vi "OE2031&OE2041_Configure Demodulation.vi"(7 "OE2041_Configure Demodulator":T1={"A"=1, "F1"=1.0, "B"=1, "F2"=1.0, "Demodulator"=1, "Mode"=0, "Arbitrary Frequency"=1000.0, "Harmonic"=1, "Instrument Mode "=8} {"Instrument Mode" items=["OE2031-10M"=6, "OE2041-30M"=7, "OE2041-60M"=8]; "Harmonic" min=1 max=32767; "Arbitrary Frequency" min=1e-05 max=60000000.0 format="%#.3f"; "Mode" items=["Harm", "Arb_Freq", "Equation"]; "Demodulator" items=["1", "2", "3"]; "F2" min=1e-05 max=60000000.0 format="%#.3g"; "B" min=-32767; "F1" min=1e-05 max=60000000.0 format="%#.3g"; "A" min=-32767}, 8 "Error in (no error)":errorcluster caption="error out（no error）", 9 "Remote Mode":u16(ring) items=["USB"=0, "RS232"=1, "Ethernet"=3], 10 "Connection ID in":refnum<k5>, 11 "VISA resource name":refnum<visa-resource-name>) -> (0 "Error out":errorcluster caption="error out", 1 "Output String":string, 2 "Connection ID out":refnum<k5>, 3 "VISA resource  out":refnum<visa-resource-name>)   [LabVIEW 2011]
panel:
  out "Demodulator":string
  # "Configure \nDemodulator  and Mode"
  # "Configure \nArbitrary Frequency"
  # "Configure Harmonic"
  # "Configure Equation"
  # "E   ="
  # "×"
  # "+"
  # "×"
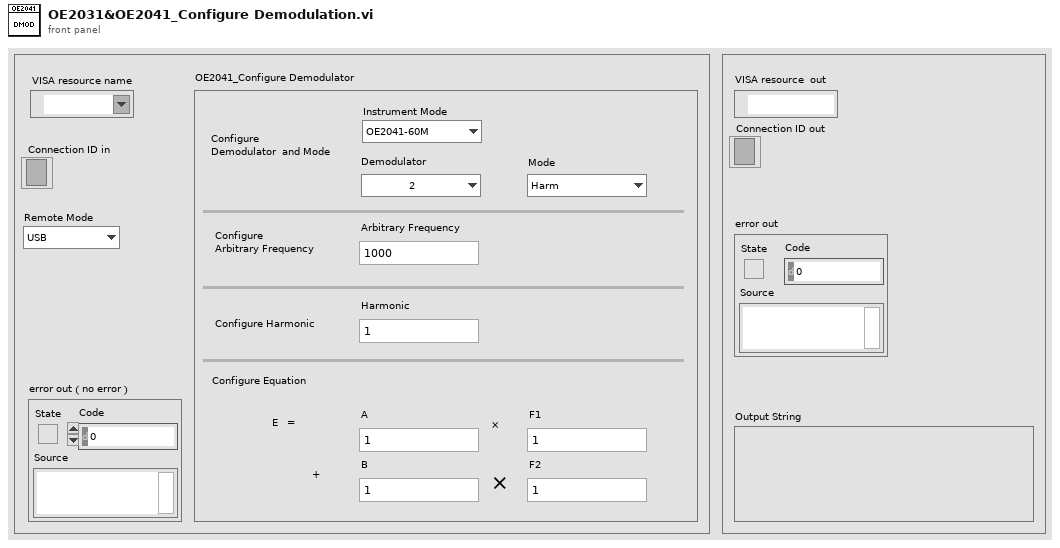
[diagram p1: front panel]
types:
  T1 = cluster{"A":i16, "F1":dbl, "B":i16, "F2":dbl, "Demodulator":u16, "Mode":u16, "Arbitrary Frequency":dbl, "Harmonic":u16, "Instrument Mode ":u16}
  T2 = enum16{"ISRC", "IGND", "ICPL", "ILIN", "PHAS", "FMOD", "RSLP", "FREQ", "SWPT", "SLLM", "SULM", "SSLL", "SSLG", "STLM", "SWRM", "IRNG", "SENS", "RMOD", "OFLT", "OFSL", "SYNC", "DMOD", "HARM", "DARB", "SWVT", "SLVL", "SVLL", "SVUL", "SVSL", "SVSG", "SVTM", "SVRM", "RALL", "SNAP", "OUTP", "OAUX", "COUT", "CAUX", "COFP", "CEXP", "FPOP", "OEXP", "*IDN", "*RST", "OVLD", "INOV", "GNOV", "*PLL", "SSET", "RSET", "AGAN", "APHS", "ARSV", "ASCL", "EQCD", "EQCS", "SPED", "SRAT", "SLEN", "SSLE", "STRG", "SPRM", "STRD", "PAUS", "REST", "SPTS", "TRCA", "TEMP", "RSTU", "IHNZ", "DEQU", "SADD", "ARNG", "CSPE", "ISRCD", "IGNDD", "ICPLD", "ILIND", "PHASD", "FMODD", "RSLPD", "FREQD", "SWPTD", "SLLMD", "SULMD", "SSLLD", "SSLGD", "STLMD", "SWRMD", "SENSD", "RMODD", "OFLTD", "OFSLD", "SYNCD", "HARMD", "EQCDD", "EQCSD", "SNAPD", "OUTPD", "SWVTD", "SLVLD", "SVLLD", "SVULD", "SVSLD", "SVSGD", "SVTMD", "SVRMD", "SVDCD", "ARSVD", "AGAND", "APHSD", "ASCLD", "FPOPD", "CAUXD", "OEXPD", "SPEDD", "SRATD", "SLEND", "SSLED", "STRGD", "SPRMD", "STRDD", "PAUSD", "RESTD", "SPTSD", "TRCAD", "*IDND", "*RSTD", "INOVD", "GNOVD", "*PLLD", "SSETD", "RSETD", "RALLD"}
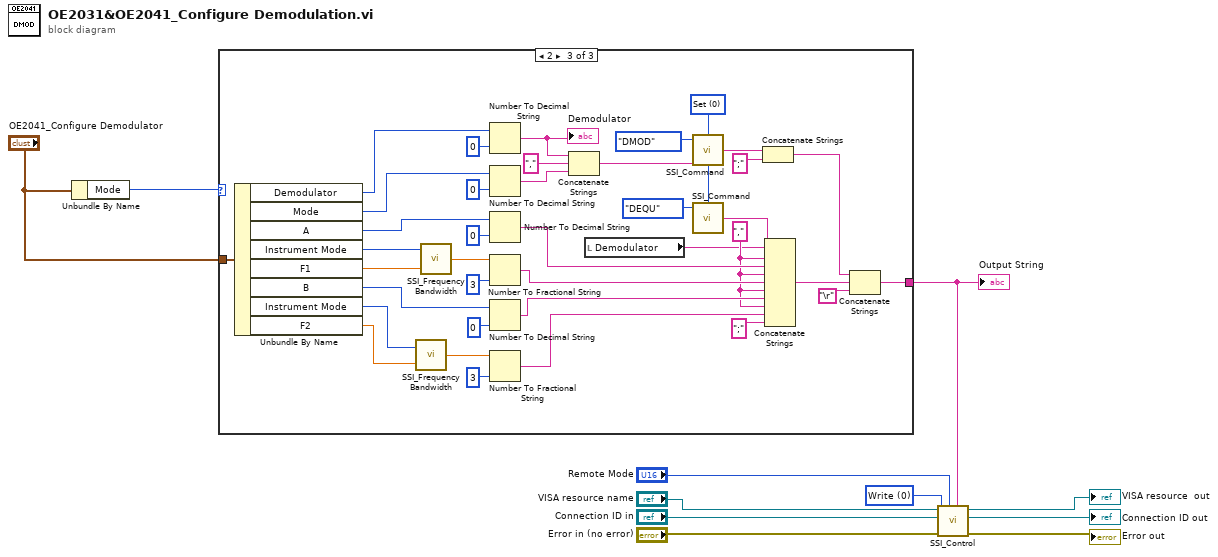
[diagram p0: block diagram]
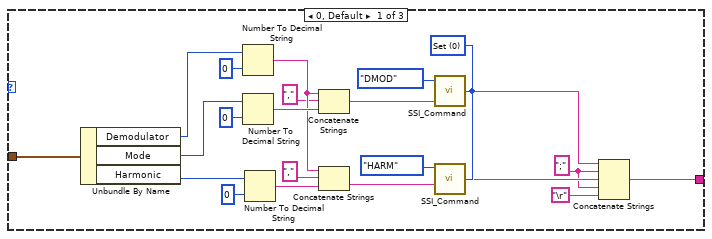
[diagram p2: hidden frame]
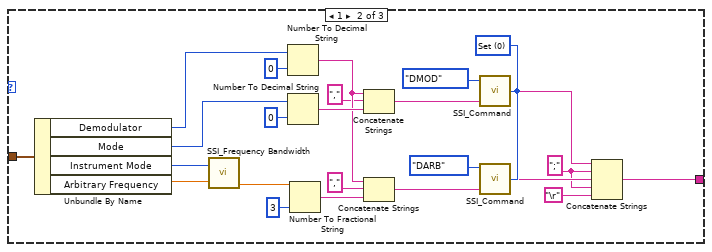
[diagram p3: hidden frame]
diagram:
  w9 = u16 0 items=["Write", "Read"] ("Control")
  n1 = Unbundle By Name("OE2041_Configure Demodulator") -> ("Mode"=w1:u16)
  n2 = case shown="2" w1 {
    tunnel: [w17 w38 w95] -> w3
    tunnel: "OE2041_Configure Demodulator" -> [w32 w37 w93]
    frame 0, Default {
      w30 = u16 0 items=["Set", "Query"] ("Opera")
      w16 = ";" ("字符串")
      n3 = Unbundle By Name(w32) -> ("Demodulator"=w28:u16, "Mode"=w23:u16, "Harmonic"=w20:u16)
      n4 = Number To Decimal String(number=w28, width (-)=i16 0 ("精度(6)")) -> (decimal integer string=w14:string)
      n5 = Number To Decimal String(number=w23, width (-)=i16 0 ("精度(6)")) -> (decimal integer string=w24:string)
      n6 = Number To Decimal String(number=w20, width (-)=i16 0 ("精度(6)")) -> (decimal integer string=w21:string)
      n7 = Concatenate Strings(w14, "," ("字符串"), w24) -> (w27:string)
      n8 = Concatenate Strings(w14, "," ("字符串"), w21) -> (w26:string)
      n9 = call "SSI_Command.vi"("Opera"=w30, "Paramter"=w27, "Command Type"=T2."DMOD") -> ("Output string"=w19:string)  [unwired: 1 in]
      n10 = call "SSI_Command.vi"("Opera"=w30, "Paramter"=w26, "Command Type"=T2."HARM") -> ("Output string"=w18:string)  [unwired: 1 in]
      n11 = Concatenate Strings(w19, w16, w18, w16, "\r") -> (w17:string)
    }
    frame 1 {
      w55 = u16 0 items=["Set", "Query"] ("Opera")
      w43 = ";" ("字符串")
      n12 = Unbundle By Name(w37) -> ("Demodulator"=w53:u16, "Mode"=w48:u16, "Instrument Mode"=w34:u16, "Arbitrary Frequency"=w35:dbl)
      n13 = call "SSI_Frequency Bandwidth.vi"("Frequency"=w35, "Instrument Mode"=w34) -> ("Output"=w36:dbl)  [unwired: 1 in]
      n14 = Number To Decimal String(number=w53, width (-)=i16 0 ("精度(6)")) -> (decimal integer string=w41:string)
      n15 = Number To Decimal String(number=w48, width (-)=i16 0 ("精度(6)")) -> (decimal integer string=w49:string)
      n16 = Number To Fractional String(number=w36, precision (6)=i16 3 ("精度(6)")) -> (F-format string=w46:string)  [unwired: 2 in]
      n17 = Concatenate Strings(w41, "," ("字符串"), w49) -> (w52:string)
      n18 = Concatenate Strings(w41, "," ("字符串"), w46) -> (w51:string)
      n19 = call "SSI_Command.vi"("Opera"=w55, "Paramter"=w52, "Command Type"=T2."DMOD") -> ("Output string"=w45:string)  [unwired: 1 in]
      n20 = call "SSI_Command.vi"("Opera"=w55, "Paramter"=w51, "Command Type"=T2."DARB") -> ("Output string"=w44:string)  [unwired: 1 in]
      n21 = Concatenate Strings(w45, w43, w44, w43, "\r") -> (w38:string)
    }
    frame 2 {
      w80 = u16 0 items=["Set", "Query"] ("Opera")
      w68 = "," ("替换字符串(\"\")")
      n22 = Unbundle By Name(w93) -> ("Demodulator"=w70:u16, "Mode"=w78:u16, "A"=w88:i16, "Instrument Mode"=w63:u16, "F1"=w62:dbl, "B"=w61:i16, "Instrument Mode"=w60:u16, "F2"=w59:dbl)
      n23 = call "SSI_Frequency Bandwidth.vi"("Frequency"=w59, "Instrument Mode"=w60) -> ("Output"=w58:dbl)  [unwired: 1 in]
      n24 = call "SSI_Frequency Bandwidth.vi"("Frequency"=w62, "Instrument Mode"=w63) -> ("Output"=w64:dbl)  [unwired: 1 in]
      n25 = Number To Decimal String(number=w70, width (-)=i16 0 ("精度(6)")) -> (decimal integer string=w69:string)
      "Demodulator" <- w69
      n26 = Number To Decimal String(number=w78, width (-)=i16 0 ("精度(6)")) -> (decimal integer string=w67:string)
      n27 = Number To Decimal String(number=w88, width (-)=i16 0 ("精度(6)")) -> (decimal integer string=w87:string)
      n28 = Number To Fractional String(number=w64, precision (6)=i16 3 ("宽度(-)")) -> (F-format string=w86:string)  [unwired: 2 in]
      n29 = Number To Decimal String(number=w61, width (-)=i16 0 ("宽度(-)")) -> (decimal integer string=w85:string)
      n30 = Number To Fractional String(number=w58, precision (6)=i16 3 ("宽度(-)")) -> (F-format string=w84:string)  [unwired: 2 in]
      n31 = Concatenate Strings(w69, "," ("字符串"), w67) -> (w74:string)
      n32 = local read "Demodulator"() -> (w65:string)
      n33 = call "SSI_Command.vi"("Opera"=w80, "Paramter"=w74, "Command Type"=T2."DMOD") -> ("Output string"=w77:string)  [unwired: 1 in]
      n34 = call "SSI_Command.vi"("Opera"=w80, "Command Type"=T2."DEQU") -> ("Output string"=w72:string)  [unwired: 2 in]
      n35 = Concatenate Strings(w77, ";" ("字符串")) -> (w75:string)
      n36 = Concatenate Strings(w72, w65, w68, w87, w68, w86, w68, w85, w68, w84, ";" ("替换字符串(\"\")")) -> (w90:string)
      n37 = Concatenate Strings(w75, w90, "\r") -> (w95:string)
    }
  }
  "Output String" <- w3
  n38 = call "SSI_Control.vi"("Write Buffer"=w3, "Remote Mode"="Remote Mode", "Error in (no error)"="Error in (no error)", "Control"=w9, "Connection ID in"="Connection ID in", "VISA resource name"="VISA resource name") -> ("Error out"=→"Error out":errorcluster, "Connection ID out"=→"Connection ID out":refnum<k5>, "VISA resource  out"=→"VISA resource  out":refnum<visa-resource-name>)  [unwired: 2 in, 1 out]
